vi "Read Analysis ROI.vi"(8 "error in (no error)":errorcluster, 11 "Analysis Graph in":refnum<class "Analysis Graph.lvclass">) -> (0 "error out":errorcluster, 2 "ROI XYZ":T1, 3 "Analysis Graph out":refnum<class "Analysis Graph.lvclass">)   [LabVIEW 2023, in "Analysis Graph.lvclass"]
uses:
  Analysis Graph.lvclass
  D:/git/Graph-Classes/source/Series Graph/Series Graph.lvclass
  D:/git/Graph-Classes/source/Base Graph/Base Graph.lvclass
  Analysis Graph.lvclass/Analysis Graph.ctl
  Base Graph/Base Graph.lvclass
  Series Graph/Series Graph.lvclass
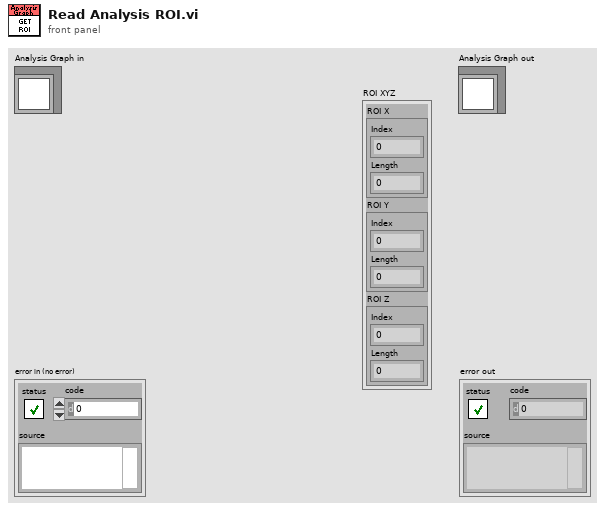
[diagram p1: front panel]
types:
  T1 = cluster{"ROI X":cluster{"Index":u32, "Length":u32}, "ROI Y":cluster{"Index":u32, "Length":u32}, "ROI Z":cluster{"Index":u32, "Length":u32}}
  T2 = cluster{"ROI X":cluster{"Index":u32, "Length":u32}, "ROI Y":cluster{"Index":u32, "Length":u32}}
  T3 = cluster{"ROI X":cluster{"Index":u32, "Length":u32}, "ROI Y":cluster{"Index":u32, "Length":u32}, "lower limit":cluster{"Index":u32, "Length":u32}}
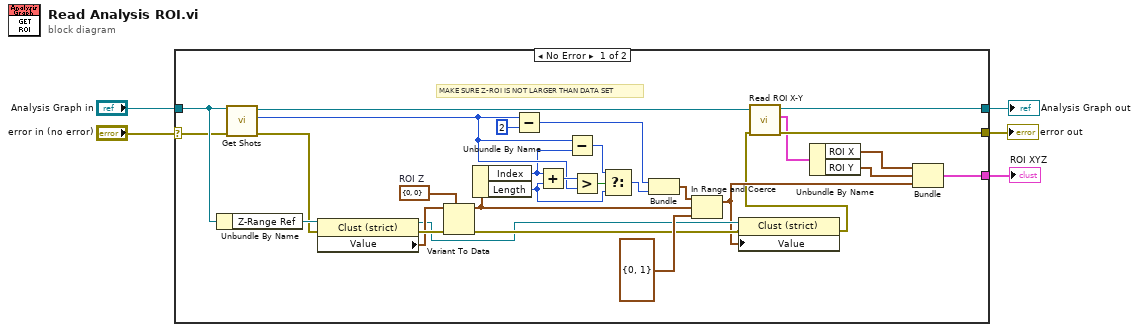
[diagram p0: block diagram]
diagram:
  n1 = case shown="No Error" "error in (no error)" {
    selector: "error in (no error)" -> [w25 w37]
    tunnel: [w33 w37] -> w4
    tunnel: [w34 w36] -> w2
    tunnel: "Analysis Graph in" -> [w26 w36]
    tunnel: [w32 _] -> w1
    frame No Error {
      w21 = cluster{"Index":u32, "Length":u32} {"Index"=0, "Length"=0}  # ROI Z
      # "MAKE SURE Z-ROI IS NOT LARGER THAN DATA SET"
      n2 = Unbundle By Name(w26) -> ("Z-Range Ref"=w35:refnum<vi>)
      n3 = call "Get Shots.vi"("error in (no error)"=w25, "Series Graph in"=w26) -> ("error out"=w22:errorcluster, "Shots"=w14:u32, "Series Graph out"=w24:refnum<class "Analysis Graph.lvclass">)  [unwired: 7 in]
      n4 = property class="Clust (strict)"(reference=w35, error in=w22) -> (reference out=w9:refnum<vi>, error out=w28:errorcluster, "Value"=w27:cluster{"Index":u32, "Length":u32})
      n5 = Variant To Data(error in=w28, type=w21, Variant=w27) -> (data=w20:cluster{"Index":u32, "Length":u32}, error out=w10:errorcluster)
      n6 = Unbundle By Name(w20) -> ("Index"=w6:u32, "Length"=w13:u32)
      n7 = Subtract(x=w14, y=u32 2) -> (x-y=w18:u32)
      n8 = Add(x=w6, y=w13) -> (x+y=w17:u32)
      n9 = Subtract(x=w14, y=w6) -> (x-y=w15:u32)
      n10 = Greater?(x=w17, y=w14) -> (0:w16:bool)
      n11 = Select(t=w15, s=w16, f=w13) -> (s? t:f=w12:u32)
      n12 = Bundle(w18, "Length"=w12) -> (w23:cluster{u32, "Length":u32})  [unwired: 1 in]
      n13 = In Range and Coerce(upper limit=w23, x=w20, lower limit=cluster{"Index":u32, "Length":u32} {"Index"=0, "Length"=1}) -> (coerced(x)=w8:cluster{"Index":u32, "Length":u32})  [unwired: 1 out]
      n14 = property class="Clust (strict)"(reference=w9, error in=w10, "Value"=w8) -> (error out=w7:errorcluster)  [unwired: 1 out]
      n15 = call "Read ROI X-Y.vi"("error in (no error)"=w7, "Base Graph in"=w24) -> ("error out"=w33:errorcluster, "ROI XY"=w31:T2, "Base Graph out"=w34:refnum<class "Analysis Graph.lvclass">)  [unwired: 7 in]
      n16 = Unbundle By Name(w31) -> ("ROI X"=w30:cluster{"Index":u32, "Length":u32}, "ROI Y"=w29:cluster{"Index":u32, "Length":u32})
      n17 = Bundle("ROI X"=w30, "ROI Y"=w29, "lower limit"=w8) -> (w32:T3)  [unwired: 1 in]
    }
    frame Error {
    }
  }
  "error out" <- w4
  "Analysis Graph out" <- w2
  "ROI XYZ" <- w1
